vi "Read Temp Cal.vi"(8 "error in (no error)":errorcluster, 11 "LINX I2C in":refnum<class "LINX I2C.lvclass">) -> (0 "error out":errorcluster, 1 "Zero":dbl, 2 "Slope":dbl, 3 "LINX I2C out":refnum<class "LINX I2C.lvclass">)   [LabVIEW 2020, in "HTS221.lvclass"]
doc: "Reads the temperature calibration values from the HTS221 device."
uses:
  HTS221.lvclass
  LINX I2C/LINX I2C.lvclass
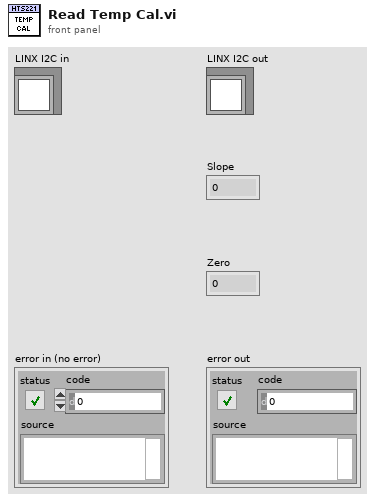
[diagram p1: front panel]
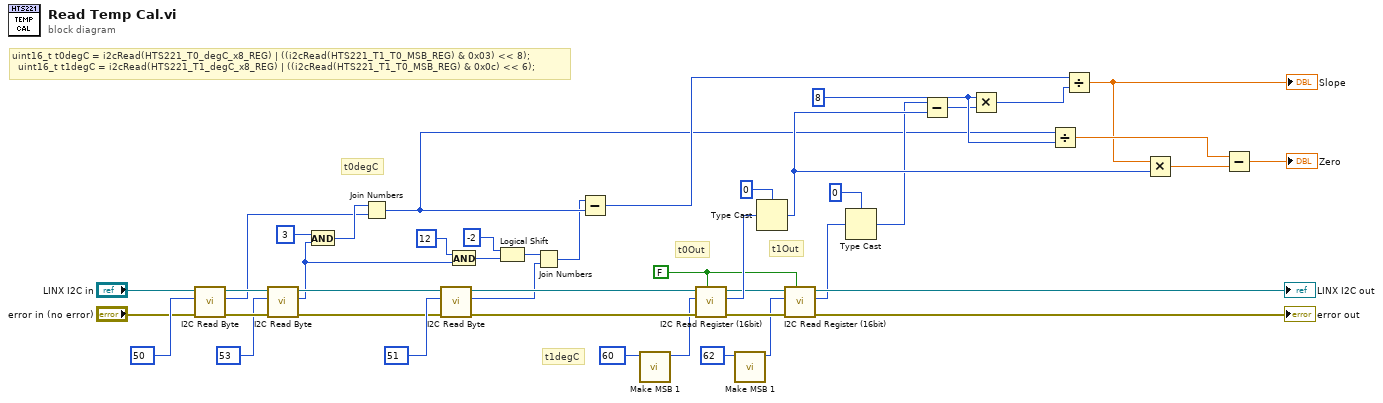
[diagram p0: block diagram]
diagram:
  w1 = FALSE ("MSB(yte) First? (T)")
  w43 = i16 8 ("x")
  # "uint16_t t0degC = i2cRead(HTS221_T0_degC_x8_REG) | ((i2cRead(HTS221_T1_T0_MSB_REG) & 0x03) << 8);\n  uint16_t t1degC = i2cRead(HTS221_T1_degC_x8_REG) | ((i2cRead(HTS221_T1_T0_MSB_REG) & 0x0c) << 6);"
  # "t1Out"
  # "t0Out"
  # "t1degC"
  # "t0degC"
  n1 = call-dynamic "I2C Read Byte.vi"("error in (no error)"="error in (no error)", "Register Address"=u8 50, "LINX I2C in"="LINX I2C in") -> ("error out"=w21:errorcluster, "Byte Read"=w15:u8, "LINX I2C out"=w19:refnum<class "LINX I2C.lvclass">)  [unwired: 6 in]
  n2 = call-dynamic "I2C Read Byte.vi"("error in (no error)"=w21, "Register Address"=u8 53, "LINX I2C in"=w19) -> ("error out"=w20:errorcluster, "Byte Read"=w12:u8, "LINX I2C out"=w18:refnum<class "LINX I2C.lvclass">)  [unwired: 6 in]
  n3 = And(x=u8 3, y=w12) -> (x .and. y?=w16:u8)
  n4 = Join Numbers(hi=w16, lo=w15) -> ((hi.lo)=w14:u16)
  n5 = call-dynamic "I2C Read Byte.vi"("error in (no error)"=w20, "Register Address"=u8 51, "LINX I2C in"=w18) -> ("error out"=w25:errorcluster, "Byte Read"=w7:u8, "LINX I2C out"=w24:refnum<class "LINX I2C.lvclass">)  [unwired: 6 in]
  n6 = And(x=u8 12, y=w12) -> (x .and. y?=w10:u8)
  n7 = Logical Shift(y=i16 -2, x=w10) -> (x << y=w8:u8)
  n8 = Join Numbers(hi=w8, lo=w7) -> ((hi.lo)=w6:u16)
  n9 = Subtract(x=w6, y=w14) -> (x-y=w32:u16)
  n10 = call "Make MSB 1.vi"("Register Address"=u8 60) -> ("Register Address | 0x80"=w4:u8)  [unwired: 10 in]
  n11 = call "I2C Read Register (16bit).vi"("MSB(yte) First? (F=Lo->Hi)"=w1, "error in (no error)"=w25, "Register Address"=w4, "LINX I2C in"=w24) -> ("error out"=w27:errorcluster, "Value"=w31:u16, "LINX I2C out"=w26:refnum<class "LINX I2C.lvclass">)  [unwired: 5 in]
  n12 = call "Make MSB 1.vi"("Register Address"=u8 62) -> ("Register Address | 0x80"=w2:u8)  [unwired: 10 in]
  n13 = Type Cast(type=i16 0, x=w31) -> (*(type *) &x=w37:i16)
  n14 = call "I2C Read Register (16bit).vi"("MSB(yte) First? (F=Lo->Hi)"=w1, "error in (no error)"=w27, "Register Address"=w2, "LINX I2C in"=w26) -> ("error out"=→"error out":errorcluster, "Value"=w28:u16, "LINX I2C out"=→"LINX I2C out":refnum<class "LINX I2C.lvclass">)  [unwired: 5 in]
  n15 = Type Cast(type=i16 0, x=w28) -> (*(type *) &x=w33:i16)
  n16 = Subtract(x=w33, y=w37) -> (x-y=w34:i16)
  n17 = Multiply(x=w43, y=w34) -> (x*y=w35:i16)
  n18 = Divide(x=w14, y=w43) -> (x/y=w39:dbl)
  n19 = Divide(x=w32, y=w35) -> (x/y=w36:dbl)
  "Slope" <- w36
  n20 = Multiply(x=w36, y=w37) -> (x*y=w38:dbl)
  n21 = Subtract(x=w39, y=w38) -> (x-y=→"Zero":dbl)
